vi "MAIN_FPGA.vi"() -> ()   [LabVIEW 2019]
uses:
  #typedef_FPGA_States.ctl
  <vilib>/Platform/TimedLoop/XDataNode/timing_clust.ctl
  <vilib>/Platform/TimedLoop/XDataNode/nitl_modes.ctl
  <vilib>/Platform/TimedLoop/XDataNode/wakeup.ctl
  #typedef_Accelerations.ctl
  <vilib>/rvi/Emulation/niFpgaGetClockAttributes.vi
  <vilib>/rvi/Emulation/niFpgaSctlEmulationGetInTimedLoop.vi
  <vilib>/rvi/Emulation/niFpgaEmulationReportErrorSimple.vi
  <vilib>/rvi/eio/common/nirviEmuTemplateMethod_errors.vi
  <vilib>/rvi/Emulation/niFpgaEmulationIsFPGAContextNoSignature.vi
  <vilib>/rvi/DataTransferAndStorage/Container/Common/niFpgaContainerGetUniqueNameForEmu.vi
  <vilib>/rvi/Memory/Memory_Emulation/niFpgaMemoryEmulationCacheClearOnFirstRun.vi
  <vilib>/rvi/Memory/Memory_Emulation/nirvimemoryEmulationManagerCache_MakeExclusive.vi
  <vilib>/rvi/Memory/Memory_Emulation/niFpgaMemoryEmulationValidateCache.vi
  <vilib>/rvi/Memory/Memory_Emulation/nirvimemoryEmulationManagerCache_InsertValue.vi
  <vilib>/Utility/error.llb/Clear Errors.vi
  <vilib>/rvi/Memory/Memory_Emulation/nirvimemoryEmulationManagerCache_ReleaseExclusive.vi
  <vilib>/rvi/Memory/Memory_Emulation/nirvimemoryEmulationManagerCache_GetValue.vi
  <vilib>/rvi/Memory/Memory_Emulation/nirvimemoryEmulationManagerCache_SetValue.vi
  <vilib>/rvi/Emulation/niFpgaProcessEmulError.vi
  <vilib>/rvi/Emulation/niFpgaCriticalErrorInLSC.vi
  <vilib>/rvi/errors/niFpgaSetErrorForExecOnDevCompSimple.vi
  <vilib>/rvi/eio/common/nirviEmuReportErrorAndStop.vi
  <vilib>/rvi/FIFO/Fifo_Resource/nirvififoEmulationSetSize.vi
  <vilib>/rvi/FIFO/Fifo_Resource/nirviFifoEmulationQueueMgr.vi
  <instcachedir>/0/nirviFifoEmulationQueueMgr_E5CAEC123FF24DC58D834DCA3CDAA9B5.lvgen/nirviFifoEmulationQueueMgr_E5CAEC123FF24DC58D834DCA3CDAA9B5_002.vi
  <vilib>/rvi/FIFO/Fifo_Resource/nirvififoEmulationDetermineInputValidOut.vi
  <vilib>/rvi/FIFO/Fifo_Resource/nirvififoEmulationCreateLock.vi
  <vilib>/rvi/FIFO/Fifo_Resource/nirvififoEmulationObtainLock.vi
  <vilib>/rvi/FIFO/Fifo_Resource/nirvififoEmulationReleaseLock.vi
  <vilib>/rvi/occurrence/nirviWaitOnOccurrenceBase.vi
  <vilib>/rvi/errors/nirviReportUnexpectedCaseInternalError.vi
  <vilib>/rvi/errors/nirviReportUnexpectedCaseInternalError (U32).vi
  <vilib>/rvi/Memory/Memory_Emulation/nirvimemoryFastEmulation.vi
  <vilib>/rvi/Memory/Memory_Emulation/nirvimemoryEmulation.vi
  <vilib>/rvi/interface/RandomDataEmulation/niFpgaRandomDataHandleErrors.vi
  <vilib>/platform/TimedLoop/XDataNode/XDataNode.xnode
  <vilib>/eio/EIONode/EIONode.xnode
  <vilib>/rvi/DataTransferAndStorage/Container/XNode/niFpgaContainer.xnode
  <vilib>/rvi/DataTransferAndStorage/Register/Emulation/niFpgaRegisterEmulation.vi
  <vilib>/rvi/FIFO/Fifo_Resource/nirvififoEmulationWrite.vi
  <vilib>/rvi/DataTransferAndStorage/Handshake/Emulation/niFpgaHandshakeEmulation.vi
  <vilib>/rvi/FIFO/Fifo_Resource/nirvififoEmulationRead.vi
  <vilib>/rvi/interface/RandomDataEmulation/nirviRandomDataFpgaReadWriteTemplate.vi
  <vilib>/Platform/TimedLoop/XDataNode/XDNodeRunTimeDep.lvlib
panel:
  out "LatestAccTimeout":bool
  in  "Monitoring?":bool
  in  "PretriggerLenght":u16
  in  "PosttriggerLenght":u16
  in  "TriggerX":i16
  in  "SamplesOverTreshold":u8
  in  "TriggerY":i16
  in  "TriggerZ":i16
  in  "stop":bool
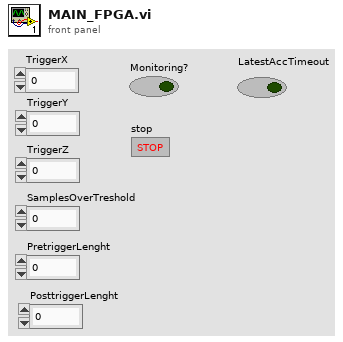
[diagram p1: front panel]
types:
  T1 = typedef "#typedef_FPGA_States.ctl" = enum16{"Idle", "Monitoring", "SendPretriggerData", "SendPostriggerData"}
  T2 = typedef "XDNodeRunTimeDep.lvlib/timing_clust.ctl" = cluster{"Expected End [f-1]":u64, "Actual End [f-1]":u64, "Finished Late? [f-1]":bool, "Expected End [i-1]":u64, "Actual End [i-1]":u64, "Finished Late? [i-1]":bool, "Expected Start [i]":u64, "Actual Start [i]":u64, "Expected Start [f]":u64, "Actual Start [f]":u64, "Source Name":string, "Structure Name":string, "Period":i64, "Deadline":i64, "Offset":i64, "Start":i64, "Priority":i32, "Timeout":i32, "Mode":T3, "Wakeup Reason":T4, "Error":errorcluster, "Source Type":string, "Secondary Source Type":string, "Global End Time":u64, "Global Start Time":u64, "Frame Duration":u64, "Iteration Duration":u64, "Assigned CPU":i32, "I/O Scan Engine Mode":u32}
  T3 = typedef "XDNodeRunTimeDep.lvlib/nitl_modes.ctl" = enum32{"No Change", "Process missed periods, maintain original phase", "Discard missed periods, maintain original phase", "Process missed periods, ignore original phase", "Discard missed periods, ignore original phase"}
  T4 = typedef "XDNodeRunTimeDep.lvlib/wakeup.ctl" = enum32{"Normal", "Aborted", "Asynchronous wakeup", "Timing source error", "Timed loop error", "Timeout"}
  T5 = cluster{"AccelerationX":i16, "AccelerationY":i16, "AccelerationZ":i16}
  T6 = typedef "#typedef_Accelerations.ctl" = cluster{"AccelerationX":i16, "AccelerationY":i16, "AccelerationZ":i16}
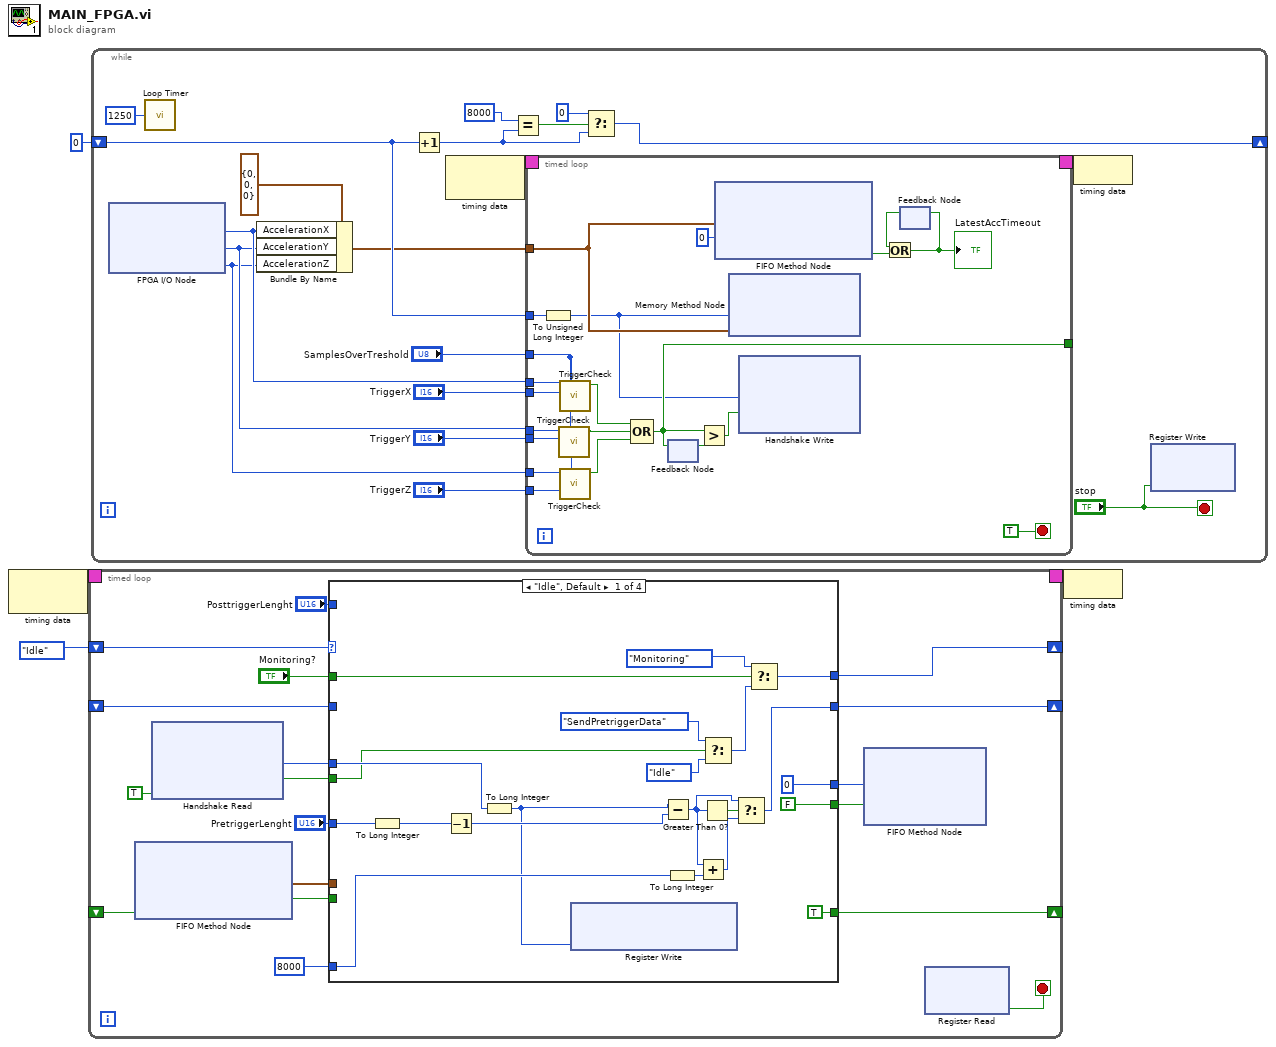
[diagram p0: block diagram]
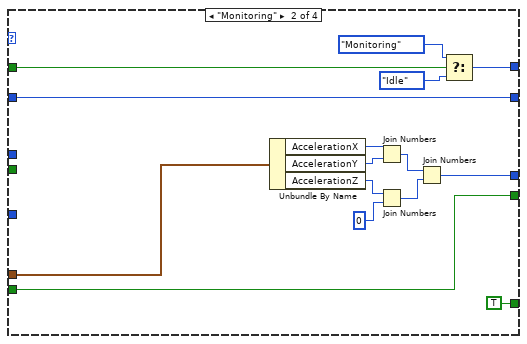
[diagram p2: hidden frame]
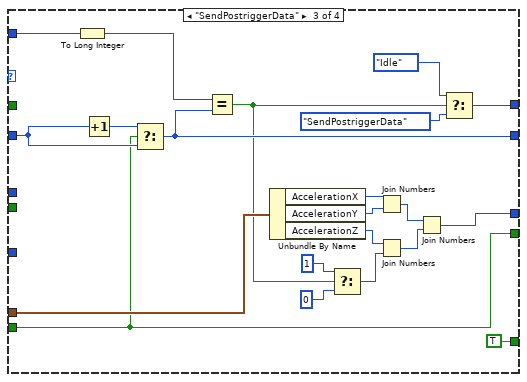
[diagram p3: hidden frame]
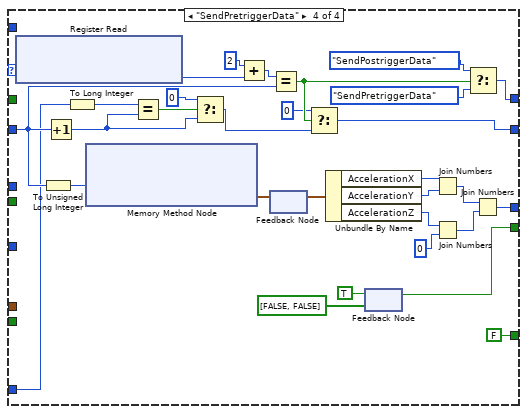
[diagram p4: hidden frame]
diagram:
  n1 = node-c288() -> (w4:T2)  [unwired: 1 in]
  n2 = timed-loop {
    timing: w4 -> [_]
    timing-out: [_] -> w3
    shift-right: [w21] -> _
    shift-left: #typedef_FPGA_States."Idle" ("FPGA States") -> [w22]
    shift-right: [w18] -> _
    shift-left: _ -> [w19]
    shift-right: [w13] -> _
    shift-left: _ -> [w14]
    stop <- w6 stop-if-true
    n3 = xnode ("FIFO Method Node")("Ready for Output"=w14) -> ("Element"=w15:T5, "Output Valid"=w12:bool)  [unwired: 1 in, 1 out]
    n4 = xnode ("Handshake Read")("Ready for Output"=TRUE) -> ("Data"=w9:u32, "Output Valid"=w10:bool)  [unwired: 1 in, 1 out]
    n5 = case shown="\"Idle\", Default" w22 {
      tunnel: [w43 w50 w72 w101] -> w21
      tunnel: [u64 0 ("Element") w51 w73 w103] -> w8
      tunnel: [FALSE ("Input Valid") w47 w64 w91] -> w7
      tunnel: "Monitoring?" -> [w39 w58 _ _]
      tunnel: w19 -> [_ w49 w65 w99]
      tunnel: [w31 w49 w66 w87] -> w18
      tunnel: "PretriggerLenght" -> [w38 _ _ _]
      tunnel: "PosttriggerLenght" -> [_ _ w71 _]
      tunnel: w15 -> [_ w48 w68 _]
      tunnel: w12 -> [_ w47 w64 _]
      tunnel: [TRUE TRUE TRUE FALSE] -> w13
      tunnel: w10 -> [w24 _ _ _]
      tunnel: w9 -> [w35 _ _ _]
      tunnel: i16 8000 -> [w28 _ _ w84]
      frame "Idle", Default {
        n6 = To Long Integer(number=w38) -> (32bit integer=w37:i32)
        n7 = Decrement(x=w37) -> (x-1=w30:i32)
        n8 = To Long Integer(number=w35) -> (32bit integer=w27:i32)
        n9 = xnode ("Register Write")("Data"=w27) -> ()  [unwired: 1 in, 1 out]
        n10 = Subtract(x=w27, y=w30) -> (x-y=w34:i32)
        n11 = To Long Integer(number=w28) -> (32bit integer=w29:i32)
        n12 = Add(x=w34, y=w29) -> (x+y=w33:i32)
        n13 = Greater Than 0?(x=w34) -> (x > 0?=w32:bool)
        n14 = Select(t=#typedef_FPGA_States."SendPretriggerData" ("FPGA States"), s=w24, f=#typedef_FPGA_States."Idle" ("FPGA States")) -> (s? t:f=w42:T1)
        n15 = Select(t=w34, s=w32, f=w33) -> (s? t:f=w31:i32)
        n16 = Select(t=#typedef_FPGA_States."Monitoring" ("FPGA States"), s=w39, f=w42) -> (s? t:f=w43:T1)
      }
      frame "Monitoring" {
        n17 = Unbundle By Name(w48) -> ("AccelerationX"=w57:i16, "AccelerationY"=w56:i16, "AccelerationZ"=w55:i16)
        n18 = Join Numbers(hi=w57, lo=w56) -> ((hi.lo)=w53:u32)
        n19 = Join Numbers(hi=w55, lo=i16 0) -> ((hi.lo)=w52:u32)
        n20 = Join Numbers(hi=w53, lo=w52) -> ((hi.lo)=w51:u64)
        n21 = Select(t=#typedef_FPGA_States."Monitoring" ("FPGA States"), s=w58, f=#typedef_FPGA_States."Idle" ("FPGA States")) -> (s? t:f=w50:T1)
      }
      frame "SendPostriggerData" {
        n22 = To Long Integer(number=w71) -> (32bit integer=w70:i32)
        n23 = Increment(x=w65) -> (x+1=w69:i32)
        n24 = Select(t=w69, s=w64, f=w65) -> (s? t:f=w66:i32)
        n25 = Equal?(x=w70, y=w66) -> (x = y?=w61:bool)
        n26 = Unbundle By Name(w68) -> ("AccelerationX"=w79:i16, "AccelerationY"=w78:i16, "AccelerationZ"=w77:i16)
        n27 = Select(t=i16 1, s=w61, f=i16 0 ("lo")) -> (s? t:f=w63:i16)
        n28 = Join Numbers(hi=w79, lo=w78) -> ((hi.lo)=w75:u32)
        n29 = Join Numbers(hi=w77, lo=w63) -> ((hi.lo)=w74:u32)
        n30 = Join Numbers(hi=w75, lo=w74) -> ((hi.lo)=w73:u64)
        n31 = Select(t=#typedef_FPGA_States."Idle" ("FPGA States"), s=w61, f=#typedef_FPGA_States."SendPostriggerData" ("FPGA States")) -> (s? t:f=w72:T1)
      }
      frame "SendPretriggerData" {
        n32 = xnode ("Register Read")() -> ("Data"=w82:i32)  [unwired: 1 in, 1 out]
        n33 = To Unsigned Long Integer(number=w99) -> (unsigned 32bit integer=w100:u32)
        n34 = Increment(x=w99) -> (x+1=w97:i32)
        n35 = To Long Integer(number=w84) -> (32bit integer=w83:i32)
        n36 = xnode ("Memory Method Node")("Address"=w100) -> ("Data"=w102:T5)  [unwired: 1 in, 1 out]
        n37 = Equal?(x=w83, y=w97) -> (x = y?=w98:bool)
        n38 = Select(t=0, s=w98, f=w97) -> (s? t:f=w96:i32)
        n39 = Add(x=2, y=w82) -> (x+y=w90:i32)
        n40 = feedback-in #1(w102) -> ()
        n41 = feedback #1() -> (w94:T5)  [unwired: 1 in]
        n42 = Equal?(x=w90, y=w99) -> (x = y?=w86:bool)
        n43 = Select(t=0, s=w86, f=w96) -> (s? t:f=w87:i32)
        n44 = Unbundle By Name(w94) -> ("AccelerationX"=w109:i16, "AccelerationY"=w108:i16, "AccelerationZ"=w107:i16)
        n45 = feedback #2(bool[] [FALSE, FALSE]) -> (w91:bool)
        n46 = feedback-in #2(TRUE) -> ()
        n47 = Join Numbers(hi=w109, lo=w108) -> ((hi.lo)=w105:u32)
        n48 = Join Numbers(hi=w107, lo=i16 0) -> ((hi.lo)=w104:u32)
        n49 = Select(t=#typedef_FPGA_States."SendPostriggerData" ("FPGA States"), s=w86, f=#typedef_FPGA_States."SendPretriggerData" ("FPGA States")) -> (s? t:f=w101:T1)
        n50 = Join Numbers(hi=w105, lo=w104) -> ((hi.lo)=w103:u64)
      }
    }
    n51 = xnode ("FIFO Method Node")("Element"=w8, "Input Valid"=w7) -> ()  [unwired: 1 in, 2 out]
    n52 = xnode ("Register Read")() -> ("Data"=w6:bool)  [unwired: 1 in, 1 out]
  }
  n53 = while {
    shift-right: [w126] -> _
    shift-left: u32 0 ("x") -> [w125]
    stop <- "stop" stop-if-true
    n54 = xnode "FPGA I/O Node"() -> ("AccelerationX"=w117:i16, "AccelerationY"=w116:i16, "AccelerationZ"=w112:i16)  [unwired: 3 in, 3 out]
    n55 = call "Loop Timer"("Count(uSec)"=u16 1250) -> ()  [unwired: 1 out]
    n56 = Bundle By Name(cluster=T6 {"AccelerationX"=0, "AccelerationY"=0, "AccelerationZ"=0} ("Accelerations"), "AccelerationX"=w117, "AccelerationY"=w116, "AccelerationZ"=w112) -> (w120:T6)
    n57 = Increment(x=w125) -> (x+1=w127:u32)
    n58 = node-c288() -> (w119:T2)  [unwired: 1 in]
    n59 = Equal?(x=u32 8000, y=w127) -> (x = y?=w129:bool)
    n60 = timed-loop {
      timing: w119 -> [_]
      timing-out: [_] -> w118
      tunnel: w125 -> [w151]
      tunnel: "SamplesOverTreshold" -> [w135]
      tunnel: w117 -> [w140]
      tunnel: w116 -> [w137]
      tunnel: "TriggerX" -> [w139]
      tunnel: "TriggerY" -> [w136]
      tunnel: "TriggerZ" -> [w134]
      tunnel: w120 -> [w146]
      tunnel: [w148] -> _
      tunnel: w112 -> [w133]
      stop <- TRUE stop-if-true
      n61 = To Unsigned Long Integer(number=w151) -> (unsigned 32bit integer=w145:u32)
      n62 = call "TriggerCheck.vi"("SamplesOverThreshold"=w135, "TriggerLevel"=w136, "Acceleration"=w137) -> ("Trigger?"=w132:bool)  [unwired: 8 in]
      n63 = call "TriggerCheck.vi"("SamplesOverThreshold"=w135, "TriggerLevel"=w139, "Acceleration"=w140) -> ("Trigger?"=w138:bool)  [unwired: 8 in]
      n64 = call "TriggerCheck.vi"("SamplesOverThreshold"=w135, "TriggerLevel"=w134, "Acceleration"=w133) -> ("Trigger?"=w131:bool)  [unwired: 8 in]
      n65 = Compound Arithmetic op=OR(w138, w132, w131) -> (w148:bool)
      n66 = feedback-in #3(w148) -> ()
      n67 = feedback #3() -> (w149:bool)  [unwired: 1 in]
      n68 = Greater?(x=w148, y=w149) -> (0:w144:bool)
      n69 = xnode ("FIFO Method Node")("Element"=w146, "Timeout"=0) -> ("Timed Out?"=w143:bool)  [unwired: 1 in, 1 out]
      n70 = xnode ("Memory Method Node")("Address"=w145, "Data"=w146) -> ()  [unwired: 1 in, 1 out]
      n71 = xnode ("Handshake Write")("Data"=w145, "Input Valid"=w144) -> ()  [unwired: 1 in, 2 out]
      n72 = feedback #4() -> (w142:bool)  [unwired: 1 in]
      n73 = Or(x=w142, y=w143) -> (x .or. y?=w141:bool)
      "LatestAccTimeout" <- w141
      n74 = feedback-in #4(w141) -> ()
    }
    n75 = Select(t=u32 0 ("x"), s=w129, f=w127) -> (s? t:f=w126:u32)
    n76 = node-c288(w118) -> ()
    n77 = xnode ("Register Write")("Data"="stop") -> ()  [unwired: 1 in, 1 out]
  }
  n78 = node-c288(w3) -> ()
